vi "Check App Data File Exist Or Create It.vi"(8 "ErrorIn":errorcluster, 9 "FileName":string, 10 "FolderName":string) -> (0 "ErrorOut":errorcluster, 3 "FilePath":path)   [LabVIEW 2019]
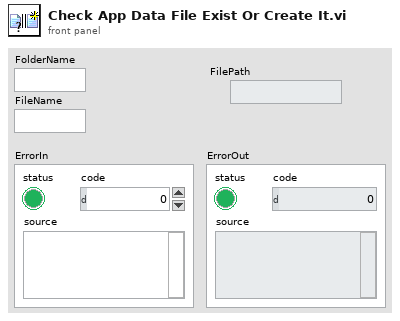
[diagram p1: front panel]
types:
  T1 = enum16{"open", "replace", "create", "open or create", "replace or create", "replace or create with confirmation"}
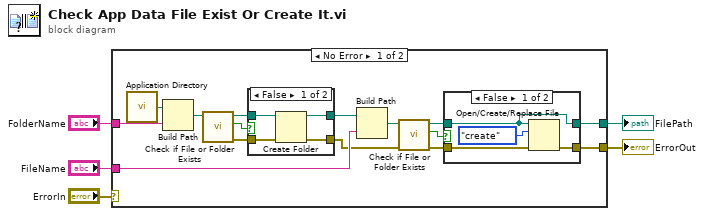
[diagram p0: block diagram]
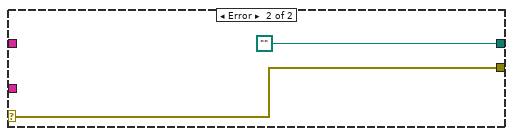
[diagram p4: hidden frame]
diagram:
  n1 = case shown="No Error" "ErrorIn" {
    selector: "ErrorIn" -> [_ w34]
    tunnel: "FolderName" -> [w19 _]
    tunnel: "FileName" -> [w18 _]
    tunnel: [w7 w34] -> w3
    tunnel: [w6 path ""] -> w2
    frame No Error {
      n2 = call <vilib>:"Application Directory.vi"() -> ("Application Directory"=w20:path)
      n3 = Build Path(base path=w20, name or relative path=w19) -> (appended path=w17:path)
      n4 = call <vilib>:"Check if File or Folder Exists.vi"("path"=w17) -> ("error out"=w14:errorcluster, "file or folder exists?"=w16:bool, "dup path"=w15:path)  [unwired: 8 in]
      n5 = case shown="False" w16 {
        tunnel: w15 -> [w30 w32]
        tunnel: w14 -> [w29 w31]
        tunnel: [w28 w31] -> w8
        tunnel: [w27 w32] -> w13
        frame False {
          n6 = Create Folder(path (use dialog)=w30, error in=w29) -> (created path=w27:path, error out=w28:errorcluster)  [unwired: 1 in, 1 out]
        }
        frame True {
        }
      }
      n7 = Build Path(base path=w13, name or relative path=w18) -> (appended path=w9:path)
      n8 = call <vilib>:"Check if File or Folder Exists.vi"("error in (no error)"=w8, "path"=w9) -> ("error out"=w12:errorcluster, "file or folder exists?"=w10:bool, "dup path"=w11:path)  [unwired: 7 in]
      n9 = case shown="False" w10 {
        tunnel: w11 -> [w21 w25]
        tunnel: w12 -> [w23 w26]
        tunnel: [w22 w26] -> w7
        tunnel: [w21 w25] -> w6
        frame False {
          n10 = Open/Create/Replace File(file path (use dialog)=w21, error in=w23, operation (0:open)=T1."create") -> (error out=w22:errorcluster)  [unwired: 3 in, 2 out]
        }
        frame True {
        }
      }
    }
    frame Error {
    }
  }
  "ErrorOut" <- w3
  "FilePath" <- w2
